vi "Caller.vi"() -> ()   [LabVIEW 2020]
panel:
  out "standard output":string
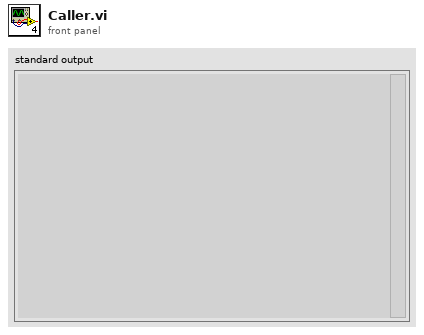
[diagram p1: front panel]
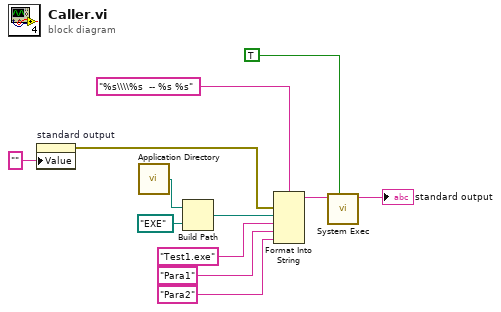
[diagram p0: block diagram]
diagram:
  n1 = property on="standard output" class="Str"("Value"="" ("standard output")) -> (error out=w2:errorcluster)  [unwired: 2 in, 1 out]
  n2 = call <vilib>:"Application Directory.vi"() -> ("Application Directory"=w12:path)
  n3 = Build Path(base path=w12, name or relative path=path "EXE") -> (appended path=w10:path)
  n4 = Format Into String(format string="%s\\\\%s  -- %s %s", error in=w2, w10, "Test1.exe", "Para1", "Para2") -> (resulting string=w6:string)  [unwired: 1 in, 1 out]
  n5 = call <vilib>:"System Exec.vi"("wait until completion? (T)"=TRUE, "command line"=w6) -> ("standard output"=→"standard output":string)  [unwired: 6 in, 3 out]
